vi "Initialize.vi"(8 "error in (no error)":errorcluster, 11 "ColorSensorDevRef":T1={"I2CDevRef"={"DevStatus"={"status"=FALSE, "code"=0, "source"=""}, "Device Address"=0, "Handle"=0, "I2C Bus"=enum."Invalid"}} {"I2CDevRef"."Device Address" format="%.0x"}) -> (0 "error out":errorcluster, 3 "ColorSensorDevRef out":T1={"I2CDevRef"={"DevStatus"={"status"=FALSE, "code"=0, "source"=""}, "Device Address"=0, "Handle"=0, "I2C Bus"=enum."Invalid"}} {"I2CDevRef"."Device Address" format="%.0x"})   [LabVIEW 2018, in "ColorSensor.lvlib"]
uses:
  ColorSensor.lvlib
  TypeDef/ColorSensorDevRef.ctl
  <vilib>/Rock Robotics/WPI/I2C/WPI_I2CDevRef.ctl
  <vilib>/Rock Robotics/SystemInterfaces/i2clib/i2c_bus.ctl
  TypeDef/LEDPulseFreq.ctl
  TypeDef/LEDCurrent.ctl
  TypeDef/ProximitySensorResolution.ctl
  TypeDef/ProximitySensorMeasurementRate.ctl
  TypeDef/ColorSensorResolution.ctl
  TypeDef/ColorSensorMeasurementRate.ctl
  TypeDef/GainFactor.ctl
  Registers.ctl
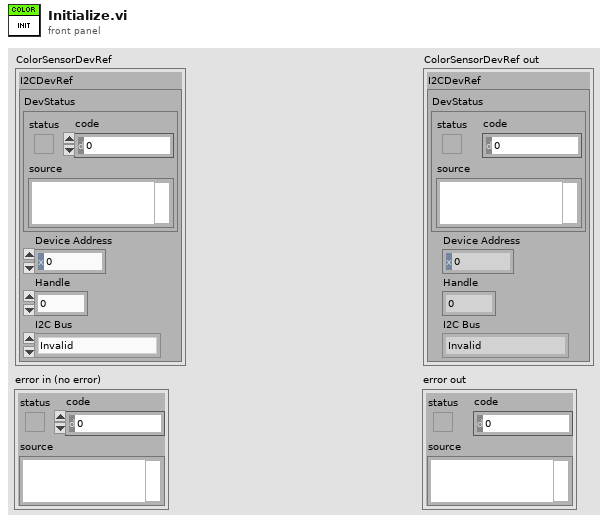
[diagram p1: front panel]
types:
  T1 = typedef "ColorSensor.lvlib/ColorSensorDevRef.ctl" = cluster{"I2CDevRef":T2}
  T2 = typedef "WPI_I2CDevRef.ctl" = cluster{"DevStatus":errorcluster, "Device Address":u8, "Handle":i32, "I2C Bus":T3}
  T3 = typedef "i2c_bus.ctl" = enum16{"I2C On-Board", "I2C MXP", "Invalid"}
  T4 = typedef "ColorSensor.lvlib/Registers.ctl" = enum16{"MainCtrl", "ProximitSensorLED", "ProximitySensorPulse", "ProximitySensorRate", "LightSensorMeasurementRate", "LightSensorGainRegister", "PartIDRegister", "MainStatus", "ProximityData", "ProximityData1", "InfraredData", "InfraredData1", "InfraredData2", "GreenData", "GreenData1", "GreenData2", "BlueData", "BlueData1", "BlueData2", "RedData", "RedData1", "RedData2"}
  T5 = typedef "ColorSensor.lvlib/GainFactor.ctl" = enum16{"1x", "3x", "6x", "9x", "18x"}
  T6 = typedef "ColorSensor.lvlib/ColorSensorMeasurementRate.ctl" = enum16{"25ms", "50ms", "100ms", "200ms", "500ms", "1000ms", "2000ms"}
  T7 = typedef "ColorSensor.lvlib/ColorSensorResolution.ctl" = enum16{"20bit", "19bit", "18bit", "17bit", "16bit", "13bit"}
  T8 = typedef "ColorSensor.lvlib/ProximitySensorMeasurementRate.ctl" = enum16{"6ms", "12ms", "25ms", "50ms", "100ms", "200ms", "400ms"}
  T9 = typedef "ColorSensor.lvlib/ProximitySensorResolution.ctl" = enum8{"8bit", "9bit", "10bit", "11bit"}
  T10 = typedef "ColorSensor.lvlib/LEDCurrent.ctl" = enum8{"2.5mA", "5.0mA", "10mA", "25mA", "50mA", "75mA", "100mA", "125mA"}
  T11 = typedef "ColorSensor.lvlib/LEDPulseFreq.ctl" = enum16{"60kHz", "70kHz", "80kHz", "90kHz", "100kHz"}
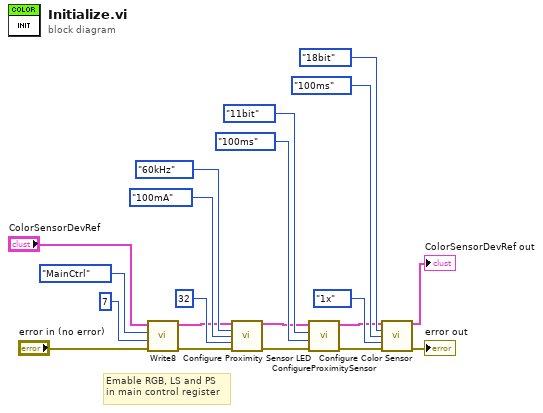
[diagram p0: block diagram]
diagram:
  # "Emable RGB, LS and PS\nin main control register"
  n1 = call "Write8.vi"("error in (no error)"="error in (no error)", "Data"=u8 7, "Registers"=Registers."MainCtrl", "ColorSensorDevRef"="ColorSensorDevRef") -> ("error out"=w1:errorcluster, "ColorSensorDevRef out"=w2:T1)  [unwired: 6 in]
  n2 = call "Configure Proximity Sensor LED.vi"("ColorSensorDevRef"=w2, "LEDPulseFreq"=LEDPulseFreq."60kHz", "LEDCurrent"=LEDCurrent."100mA", "Pulses"=u8 32, "error in (no error)"=w1) -> ("ColorSensorDevRef out"=w14:T1, "error out"=w15:errorcluster)  [unwired: 9 in]
  n3 = call "ConfigureProximitySensor.vi"("error in (no error)"=w15, "ProximitySensorMeasurementRate"=ProximitySensorMeasurementRate."100ms", "ProximitySensorResolution"=ProximitySensorResolution."11bit", "ColorSensorDevRef"=w14) -> ("error out"=w9:errorcluster, "ColorSensorDevRef out"=w10:T1)  [unwired: 6 in]
  n4 = call "Configure Color Sensor.vi"("ColorSensorDevRef"=w10, "ColorSensorResolution"=ColorSensorResolution."18bit", "ColorSensorMeasurementRate"=ColorSensorMeasurementRate."100ms", "GainFactor"=GainFactor."1x", "error in (no error)"=w9) -> ("ColorSensorDevRef out"=→"ColorSensorDevRef out":T1, "error out"=→"error out":errorcluster)  [unwired: 9 in]
